vi "Sample 1.vi"() -> ()   [LabVIEW 2026]
panel:
  out "In Range?":bool
  out "coerced(x)":dbl
  in  "lower limit":dbl
  in  "upper limit":dbl
  in  "x":dbl
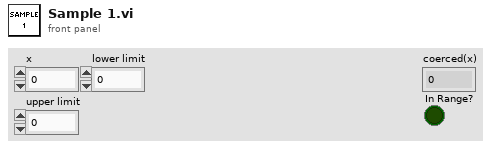
[diagram p1: front panel]
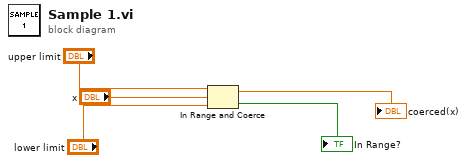
[diagram p0: block diagram]
diagram:
  n1 = In Range and Coerce(upper limit="upper limit", x="x", lower limit="lower limit") -> (coerced(x)=→"coerced(x)":dbl, In Range?=→"In Range?":bool)
